vi "Formulate VI Call Chain.vi"(5 "Call Chain":string[](array[string])) -> (6 "String Out":string)   [LabVIEW 2014, in "FH 55.lvlib"]
doc: "This VI accepts the caller VI's \"Call Chain\", which is an array of strings. It converts the string array into a string with \" -> \" between each element of the chain."
uses:
  FH 55.lvlib
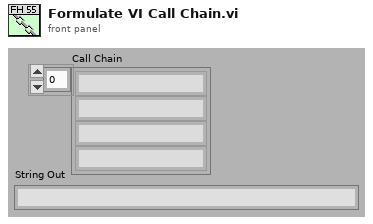
[diagram p1: front panel]
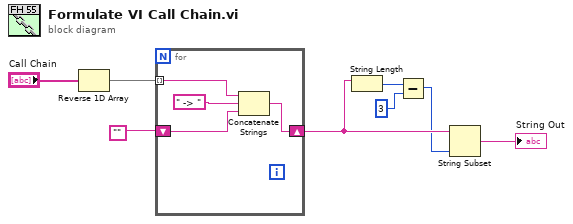
[diagram p0: block diagram]
diagram:
  n1 = Reverse 1D Array(array="Call Chain") -> (reversed array=w3:string[])
  n2 = for {
    tunnel: w3 -> [w12] mode=indexing
    shift-right: [w10] -> w5
    shift-left: "" -> [w9]
    n3 = Concatenate Strings(w12, " -> ", w9) -> (w10:string)
  }
  n4 = String Length(string=w5) -> (length=w7:i32)
  n5 = Subtract(x=w7, y=3) -> (x-y=w4:i32)
  n6 = String Subset(string=w5, length (rest)=w4) -> (substring=→"String Out":string)  [unwired: 1 in]
